vi "BFG Production Data.vi"(7 "array":dbl[][](array[numeric])) -> (8 "Threshold Values":u16[](array[numeric]))   [LabVIEW 2010]
panel:
  # "•\tBattery 75% Voltage Threshold, No Load: 3.950V\n•\tBattery 75% Voltage Threshold, Stimulation On: 3.925V\n•\tBattery 50% Voltage Threshold, No Load: 3.850V\n•\tBattery 50% Voltage Threshold, Stimulation On: 3.825V\n•\tBattery 25% Voltage Threshold, No Load: 3.780V\n•\tBattery 25% Voltage Threshold, Stimulation On: 3.755V\n•\tBattery Warning Voltage Threshold, No Load: 3.740V\n•\tBattery Warning Voltage Threshold, Stimulation On: 3.715V\n•\tBattery Critical Voltage Threshold, No Load: 3.720V\n•\tBattery Critical Voltage Threshold, Stimulation On: 3.695V\n•\tMinimum Safe Stimulating Voltage, No Load: 3.700V\n•\tMinimum Safe Stimulation Voltage, Stimulation On: 3.675V\n•\tBattery Cut-off Voltage Threshold:  2.850V"
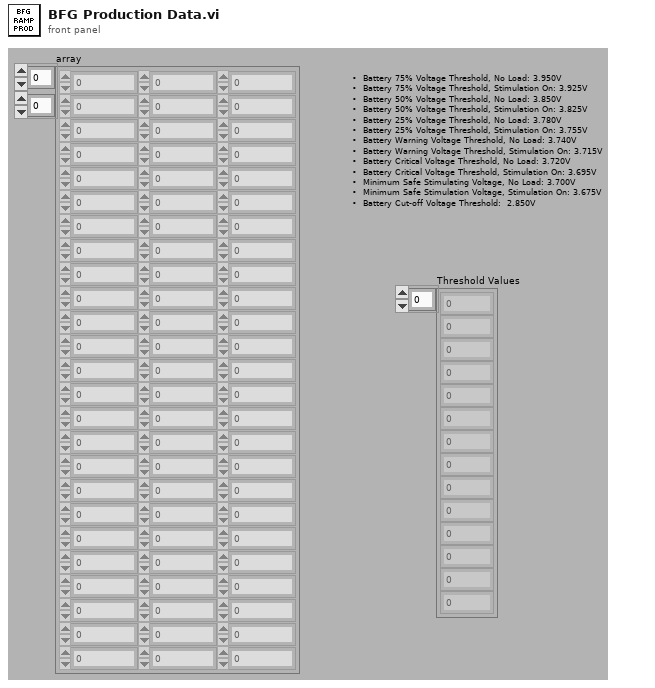
[diagram p1: front panel]
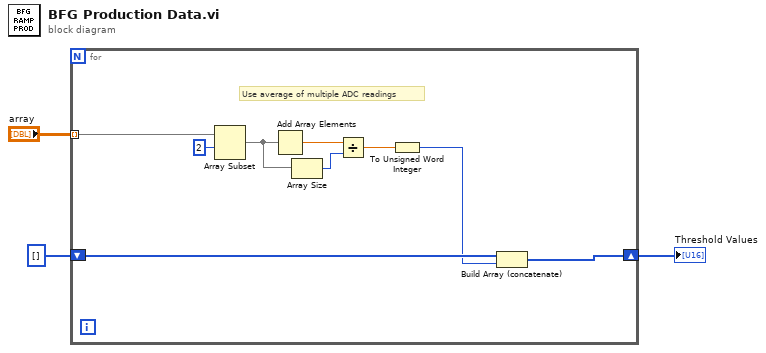
[diagram p0: block diagram]
diagram:
  n1 = for {
    shift-right: [w11] -> w3
    shift-left: u16[] [] -> [w12]
    tunnel: "array" -> [w10] mode=indexing
    # "Use average of multiple ADC readings"
    n2 = Array Subset(array=w10, index=2) -> (w7:dbl[])  [unwired: 1 in]
    n3 = Add Array Elements(numeric array=w7) -> (sum=w5:dbl)
    n4 = Array Size(array=w7) -> (size(s)=w6:i32)
    n5 = Divide(x=w5, y=w6) -> (x/y=w4:dbl)
    n6 = To Unsigned Word Integer(number=w4) -> (unsigned 16bit integer=w9:u16)
    n7 = Build Array (concatenate)(w12, w9) -> (w11:u16[])
  }
  "Threshold Values" <- w3
